vi "GUI_Single Button Pump.vi"() -> ()   [LabVIEW 2011] (continued)
                            n246 = Close Reference(reference=w680, error in (no error)=w679) -> (error out=w678:errorcluster)
                            n247 = invoke on="User Input Panel" class="SubPnl" method="Remove VI"(error in=w678) -> ()  [unwired: 2 in, 3 out]
                          }
                          frame Error {
                          }
                        }
                      }
                    }
                    n248 = call "MID-VAC Timer.vi"("TO sec (Start timer)"=1.0, "Action"=timerAction_typdef."Start Timer") -> ()  [unwired: 9 in, 1 out]
                  }
                  frame True {
                    # "when to is true\nand"
                    n249 = case shown="False" w682 {
                      tunnel: w683 -> [w689 _]
                      tunnel: [w687 w704] -> w684
                      tunnel: w681 -> [w685 w705]
                      frame False {
                        n250 = call "FindControlByName_VEPS.vi"("control name"="Op Out", "vi refnum"=w689) -> ("control refnum"=w691:refnum<vi>)  [unwired: 2 in, 1 out]
                        n251 = property class="Ctl"(reference=w691) -> ("Value"=w690:variant)  [unwired: 1 in, 2 out]
                        n252 = Variant To Data(type=op_typdef."Idle" ("Op Out"), Variant=w690) -> (data=w688:T24)  [unwired: 1 in, 1 out]
                        n253 = case shown="\"Continue to Wait\"" w688 {
                          tunnel: [w693 w699 "Idle\nMacro: Exit"] -> w687
                          tunnel: w685 -> [w694 w698 _]
                          frame "Idle", Default {
                            n254 = call "MID-VAC Timer.vi"("TO sec (Start timer)"=30.0, "Action"=timerAction_typdef."Start Timer") -> ()  [unwired: 9 in, 1 out]
                            n255 = Concatenate Strings("Main: BTL Sanity Check>>", w694) -> (w693:string)
                          }
                          frame "Continue to Wait" {
                            # "Continue to wait. Reset Timer"
                            n256 = call "MID-VAC Timer.vi"("TO sec (Start timer)"=30.0, "Action"=timerAction_typdef."Start Timer") -> ()  [unwired: 9 in, 1 out]
                            n257 = Concatenate Strings("Main: BTL Sanity Check>>", w698) -> (w699:string)
                          }
                          frame "Exit" {
                          }
                        }
                      }
                      frame True {
                        n258 = Concatenate Strings("Main: BTL Sanity Check>>", w705) -> (w704:string)
                      }
                    }
                  }
                }
                n259 = call "MID-VAC Timer.vi"("Action"=timerAction_typdef."Timer Running") -> ("TO"=w657:bool)  [unwired: 10 in]
                n260 = And(x=w652, y=w657) -> (x .and. y?=w656:bool)
                n261 = Concatenate Strings(w648, " Valve is NOT Closed. Perform corrective action.\nClick on continue to wait for some more time.\nClick Exit to abort GPM" ("message")) -> (w649:string)
                n262 = call "Generate TO event.vi"("Boolean"=w656, "message"=w649, "User Event in"=w659) -> ()  [unwired: 9 in]
              }
            }
          }
        }
        n263 = call <vilib>:"Add State(s) to Queue__jki_lib_state_machine.vi"("State(s) in Front (\"\")"=w623, "State(s) in (\"\")"=w617) -> ("States Out"=w628:string)  [unwired: 13 in]
      }
      frame "Main: TARGET Sanity Check" {
        # "Check if gate valve between COMP and M123 is Open"
        n264 = Unbundle By Name(w713) -> ("Chamber Selection.BTL"=w711:bool, "Chamber Selection.TARGET"=w712:bool, "Chamber Selection.BTL2"=w710:bool)
        n265 = case shown="True" w712 {
          tunnel: w718 -> [w721 w730]
          tunnel: w717 -> [_ w729]
          tunnel: [w721 w728] -> w716
          tunnel: w715 -> [_ w727]
          tunnel: ["" w726] -> w714
          tunnel: w713 -> [_ w725]
          tunnel: w711 -> [_ w723]
          tunnel: w710 -> [_ w722]
          tunnel: w709 -> [_ w724]
          frame False {
          }
          frame True {
            # "Check Conditions"
            n266 = case shown="\"BTL-TARGET,TARGET-BTL2\"" w724 {
              selector: w724 -> [_ w739]
              tunnel: w730 -> [w738 w756]
              tunnel: w729 -> [_ w755]
              tunnel: [w738 w753] -> w728
              tunnel: w727 -> [_ w750]
              tunnel: [w735 w744] -> w726
              tunnel: w725 -> [_ w742]
              tunnel: w723 -> [w732 _]
              tunnel: w722 -> [w736 _]
              frame "False", Default {
                # "COMP SELECTED?"
                n267 = Select(t="", s=w732, f="Main: TARGET Sanity Check>>BTL-TARGET") -> (s? t:f=w733:string)
                n268 = Select(t=w733, s=w736, f="Main: TARGET Sanity Check>>BTL-TARGET\nMain: TARGET Sanity Check>>TARGET-BTL2") -> (s? t:f=w735:string)
              }
              frame "BTL-TARGET,TARGET-BTL2" {
                w751 = Error_codes."003-Chamber Gate Valve Status" ("Error Codes")
                # "Event TAG"
                n269 = case shown="\"BTL-TARGET\"" w739 {
                  tunnel: [w758 w759 w760] -> w757
                  frame "False", Default {
                    w758 = T32[] [enum."No Action"] items=["No Action", "Is EC GPM Mode ON?", "Is EC GPM Mode Off?", "Is EC GVM Mode ON?", "Is EC GVM Off?", "Is  EC GPM or GVM Mode ON?", "Is LB GPM Mode ON?", "Is LB GPM Mode Off?", "Is LB GVM Mode ON?", "Is LB GVM Mode Off?", "Is  LB GPM or GVM Mode ON?", "Is M123 Turbo Gate Valve Opened? ", "Is M123 Turbo Gate Valve Closed?", "Is OAP Turbo Gate Valve Opened?", "Is OAP Turbo Gate Valve Closed?", "Is BTLTurbo Gate Valve Opened?", "Is BTL Turbo Gate Valve Closed?", "Is TARGET Turbo Gate Valve 1Opened?", "Is TARGET1 Turbo Gate Valve Closed?", "Is TARGET Turbo Gate Valve 2 Opened?", "Is TAREGT2 Turbo Gate Valve Closed?", "Is BTL2 Turbo Gate Valve Opened?", "Is BTL2 Turbo Gate Valve Closed?", "Is HPD Turbo Gate Valve Opened?", "Is HPD Turbo Gate Valve Closed?", "Is COMP to M123 gate Valve Opened?", "Is COMP to M123 Valve Closed?", "Is HPBD Gate Valve Opened?", "Is HPBD Gate Valve Closed?", "Is M123 to OAP gate valve opened?", "Is M123 to OAP gate valve closed?", "Is OAP to BLT gate valve opened?", "Is OAP to BTL Gate Valve Closed?", "Is BLT to TARGET gate valve opened?", "Is BTL to TARGET Gate Valve Closed?", "Is TARGET to BLT2 gate valve opened?", "Is TARGET to BTL2 Gate Valve Closed?", "Is BLT2 to HPD gate valve opened?", "Is BTL2 to HPD Gate Valve Closed?", "Is COMP at Atmospheric Pressure?", "Is M123 at Atmospheric Pressure?", "Is BeamDump at Atmospheric Pressure?", "Is OAP at Atmospheric Pressure?", "Is BLT at Atmospheric Pressure", "Is TARGET at Atmospheric Pressure?", "Is BLT2 at Atmospheric Pressure?", "Is HPD at Atmospheric Pressure?", "Is the EC Roughing Pump ON?", "Is the EC Roughing Pump OFF?", "Does the EC Roughing Pump have a fault?", "Is the LB Roughing Pump ON?", "Is the LB Roughing Pump Off?", "Does the LB Roughing Pump have a fault?", "Is the EC Backing Pump ON?", "Is the EC Backing Pump OFF?", "Is the LB Backing Pump ON?", "Is the LB Backing Pump OFF?", "Does the EC Backing Pump have a fault?", "Does the LB Backing Pump have a fault?", "Is the EC Backing Pipe at Atmospheric Pressure", "Is the LB Backing Pipe at Atmospheric Pressure", "Is the EC Backing Manifold at Atmospheric Pressure", "s the LB Backing Manifold at Atmospheric Pressure?", "Is the EC Roughing Pipe at Atmospheric Pressure", "Is the LB Roughing Pipe at Atmospheric Pressure?", "Is the EC Roughing Manifold at Atmospheric Pressure", "Is the LB Roughing Manifold at Atmospheric Pressure", "Is LB Backing Manifold Valve Opened?", "Is EC Backing Manifold Valve Opened?", "Is LB Roughing Manifold Valve Opened?", "Is EC Roughing Manifold Valve Opened?", "Is COMP Roughing Valve Opened?", "Is M123 Roughing Valve Opened?", "Is M123 Roughing Valve Closed?", "Is OAP Roughing Valve Opened?", "Is OAP Roughing Valve Closed?", "Is HPBD Roughing Valve Opened?", "Is HPBD Roughing Valve Closed?", "Is BTL Roughing Valve Opened?", "Is BTL Roughing Valve Closed?", "Is TARGET Roughing Valve Opened?", "Is TARGET Roughing Valve Closed?", "Is BTL2 Roughing Valve Opened?", "Is BTL2 Roughing Valve Closed?", "Is HPD Roughing Valve Opened?", "Is HPD Roughing Valve Closed?", "Is COMP Turbo Backing Valve Opened?", "Is M123 Turbo Backing Valve Opened", "Is HPBD Turbo Backing Valve Opened?", "Is OAP Turbo Backing Valve Opened?", "Is BTL Turbo Backing Valve Opened?", "Is TARGET1 Turbo Backing Valve Opened?", "Is TARGET2 Turbo Backing Valve Opened?", "Is BTL2 Turbo Backing Valve Opened?", "Is HPD Turbo Backing Valve Opened?", "Is M123 Backing at MID-VAC?", "Is OAP Backing at MID-VAC?", "Is TARGET1 Backing at MID-VAC?", "Is TARGET2 Backing at MID-VAC?", "Is BTL Backing at MID-VAC?", "Is BTL2 Backing at MID-VAC?", "Is HPD Backing at MID-VAC?", "Is M123 Turbo in Normal Operation", "Is COMP Turbo in Normal Operation", "Is OAP Turbo in Normal Operation", "Is BTL Turbo in Normal Operation", "Is TARGET1 Turbo in Normal Operation", "Is TARGET2 Turbo in Normal Operation", "Is BTL2 Turbo in Normal Operation", "Is HPD Turbo in Normal Operation", "Is M123 at MID-VAC?", "Is OAP at MID-VAC?", "Is COMP at MID-VAC?", "Is BTL at MID-VAC?", "Is TARGET at MID-VAC?", "Is BTL2 at MID-VAC?", "Is HPD at MID-VAC?"]
                  }
                  frame "TARGET-BTL2" {
                    w759 = T32[] [enum."Is TARGET to BTL2 Gate Valve Closed?"] items=["No Action", "Is EC GPM Mode ON?", "Is EC GPM Mode Off?", "Is EC GVM Mode ON?", "Is EC GVM Off?", "Is  EC GPM or GVM Mode ON?", "Is LB GPM Mode ON?", "Is LB GPM Mode Off?", "Is LB GVM Mode ON?", "Is LB GVM Mode Off?", "Is  LB GPM or GVM Mode ON?", "Is M123 Turbo Gate Valve Opened? ", "Is M123 Turbo Gate Valve Closed?", "Is OAP Turbo Gate Valve Opened?", "Is OAP Turbo Gate Valve Closed?", "Is BTLTurbo Gate Valve Opened?", "Is BTL Turbo Gate Valve Closed?", "Is TARGET Turbo Gate Valve 1Opened?", "Is TARGET1 Turbo Gate Valve Closed?", "Is TARGET Turbo Gate Valve 2 Opened?", "Is TAREGT2 Turbo Gate Valve Closed?", "Is BTL2 Turbo Gate Valve Opened?", "Is BTL2 Turbo Gate Valve Closed?", "Is HPD Turbo Gate Valve Opened?", "Is HPD Turbo Gate Valve Closed?", "Is COMP to M123 gate Valve Opened?", "Is COMP to M123 Valve Closed?", "Is HPBD Gate Valve Opened?", "Is HPBD Gate Valve Closed?", "Is M123 to OAP gate valve opened?", "Is M123 to OAP gate valve closed?", "Is OAP to BLT gate valve opened?", "Is OAP to BTL Gate Valve Closed?", "Is BLT to TARGET gate valve opened?", "Is BTL to TARGET Gate Valve Closed?", "Is TARGET to BLT2 gate valve opened?", "Is TARGET to BTL2 Gate Valve Closed?", "Is BLT2 to HPD gate valve opened?", "Is BTL2 to HPD Gate Valve Closed?", "Is COMP at Atmospheric Pressure?", "Is M123 at Atmospheric Pressure?", "Is BeamDump at Atmospheric Pressure?", "Is OAP at Atmospheric Pressure?", "Is BLT at Atmospheric Pressure", "Is TARGET at Atmospheric Pressure?", "Is BLT2 at Atmospheric Pressure?", "Is HPD at Atmospheric Pressure?", "Is the EC Roughing Pump ON?", "Is the EC Roughing Pump OFF?", "Does the EC Roughing Pump have a fault?", "Is the LB Roughing Pump ON?", "Is the LB Roughing Pump Off?", "Does the LB Roughing Pump have a fault?", "Is the EC Backing Pump ON?", "Is the EC Backing Pump OFF?", "Is the LB Backing Pump ON?", "Is the LB Backing Pump OFF?", "Does the EC Backing Pump have a fault?", "Does the LB Backing Pump have a fault?", "Is the EC Backing Pipe at Atmospheric Pressure", "Is the LB Backing Pipe at Atmospheric Pressure", "Is the EC Backing Manifold at Atmospheric Pressure", "s the LB Backing Manifold at Atmospheric Pressure?", "Is the EC Roughing Pipe at Atmospheric Pressure", "Is the LB Roughing Pipe at Atmospheric Pressure?", "Is the EC Roughing Manifold at Atmospheric Pressure", "Is the LB Roughing Manifold at Atmospheric Pressure", "Is LB Backing Manifold Valve Opened?", "Is EC Backing Manifold Valve Opened?", "Is LB Roughing Manifold Valve Opened?", "Is EC Roughing Manifold Valve Opened?", "Is COMP Roughing Valve Opened?", "Is M123 Roughing Valve Opened?", "Is M123 Roughing Valve Closed?", "Is OAP Roughing Valve Opened?", "Is OAP Roughing Valve Closed?", "Is HPBD Roughing Valve Opened?", "Is HPBD Roughing Valve Closed?", "Is BTL Roughing Valve Opened?", "Is BTL Roughing Valve Closed?", "Is TARGET Roughing Valve Opened?", "Is TARGET Roughing Valve Closed?", "Is BTL2 Roughing Valve Opened?", "Is BTL2 Roughing Valve Closed?", "Is HPD Roughing Valve Opened?", "Is HPD Roughing Valve Closed?", "Is COMP Turbo Backing Valve Opened?", "Is M123 Turbo Backing Valve Opened", "Is HPBD Turbo Backing Valve Opened?", "Is OAP Turbo Backing Valve Opened?", "Is BTL Turbo Backing Valve Opened?", "Is TARGET1 Turbo Backing Valve Opened?", "Is TARGET2 Turbo Backing Valve Opened?", "Is BTL2 Turbo Backing Valve Opened?", "Is HPD Turbo Backing Valve Opened?", "Is M123 Backing at MID-VAC?", "Is OAP Backing at MID-VAC?", "Is TARGET1 Backing at MID-VAC?", "Is TARGET2 Backing at MID-VAC?", "Is BTL Backing at MID-VAC?", "Is BTL2 Backing at MID-VAC?", "Is HPD Backing at MID-VAC?", "Is M123 Turbo in Normal Operation", "Is COMP Turbo in Normal Operation", "Is OAP Turbo in Normal Operation", "Is BTL Turbo in Normal Operation", "Is TARGET1 Turbo in Normal Operation", "Is TARGET2 Turbo in Normal Operation", "Is BTL2 Turbo in Normal Operation", "Is HPD Turbo in Normal Operation", "Is M123 at MID-VAC?", "Is OAP at MID-VAC?", "Is COMP at MID-VAC?", "Is BTL at MID-VAC?", "Is TARGET at MID-VAC?", "Is BTL2 at MID-VAC?", "Is HPD at MID-VAC?"]
                  }
                  frame "BTL-TARGET" {
                    w760 = T32[] [enum."Is BTL to TARGET Gate Valve Closed?"] items=["No Action", "Is EC GPM Mode ON?", "Is EC GPM Mode Off?", "Is EC GVM Mode ON?", "Is EC GVM Off?", "Is  EC GPM or GVM Mode ON?", "Is LB GPM Mode ON?", "Is LB GPM Mode Off?", "Is LB GVM Mode ON?", "Is LB GVM Mode Off?", "Is  LB GPM or GVM Mode ON?", "Is M123 Turbo Gate Valve Opened? ", "Is M123 Turbo Gate Valve Closed?", "Is OAP Turbo Gate Valve Opened?", "Is OAP Turbo Gate Valve Closed?", "Is BTLTurbo Gate Valve Opened?", "Is BTL Turbo Gate Valve Closed?", "Is TARGET Turbo Gate Valve 1Opened?", "Is TARGET1 Turbo Gate Valve Closed?", "Is TARGET Turbo Gate Valve 2 Opened?", "Is TAREGT2 Turbo Gate Valve Closed?", "Is BTL2 Turbo Gate Valve Opened?", "Is BTL2 Turbo Gate Valve Closed?", "Is HPD Turbo Gate Valve Opened?", "Is HPD Turbo Gate Valve Closed?", "Is COMP to M123 gate Valve Opened?", "Is COMP to M123 Valve Closed?", "Is HPBD Gate Valve Opened?", "Is HPBD Gate Valve Closed?", "Is M123 to OAP gate valve opened?", "Is M123 to OAP gate valve closed?", "Is OAP to BLT gate valve opened?", "Is OAP to BTL Gate Valve Closed?", "Is BLT to TARGET gate valve opened?", "Is BTL to TARGET Gate Valve Closed?", "Is TARGET to BLT2 gate valve opened?", "Is TARGET to BTL2 Gate Valve Closed?", "Is BLT2 to HPD gate valve opened?", "Is BTL2 to HPD Gate Valve Closed?", "Is COMP at Atmospheric Pressure?", "Is M123 at Atmospheric Pressure?", "Is BeamDump at Atmospheric Pressure?", "Is OAP at Atmospheric Pressure?", "Is BLT at Atmospheric Pressure", "Is TARGET at Atmospheric Pressure?", "Is BLT2 at Atmospheric Pressure?", "Is HPD at Atmospheric Pressure?", "Is the EC Roughing Pump ON?", "Is the EC Roughing Pump OFF?", "Does the EC Roughing Pump have a fault?", "Is the LB Roughing Pump ON?", "Is the LB Roughing Pump Off?", "Does the LB Roughing Pump have a fault?", "Is the EC Backing Pump ON?", "Is the EC Backing Pump OFF?", "Is the LB Backing Pump ON?", "Is the LB Backing Pump OFF?", "Does the EC Backing Pump have a fault?", "Does the LB Backing Pump have a fault?", "Is the EC Backing Pipe at Atmospheric Pressure", "Is the LB Backing Pipe at Atmospheric Pressure", "Is the EC Backing Manifold at Atmospheric Pressure", "s the LB Backing Manifold at Atmospheric Pressure?", "Is the EC Roughing Pipe at Atmospheric Pressure", "Is the LB Roughing Pipe at Atmospheric Pressure?", "Is the EC Roughing Manifold at Atmospheric Pressure", "Is the LB Roughing Manifold at Atmospheric Pressure", "Is LB Backing Manifold Valve Opened?", "Is EC Backing Manifold Valve Opened?", "Is LB Roughing Manifold Valve Opened?", "Is EC Roughing Manifold Valve Opened?", "Is COMP Roughing Valve Opened?", "Is M123 Roughing Valve Opened?", "Is M123 Roughing Valve Closed?", "Is OAP Roughing Valve Opened?", "Is OAP Roughing Valve Closed?", "Is HPBD Roughing Valve Opened?", "Is HPBD Roughing Valve Closed?", "Is BTL Roughing Valve Opened?", "Is BTL Roughing Valve Closed?", "Is TARGET Roughing Valve Opened?", "Is TARGET Roughing Valve Closed?", "Is BTL2 Roughing Valve Opened?", "Is BTL2 Roughing Valve Closed?", "Is HPD Roughing Valve Opened?", "Is HPD Roughing Valve Closed?", "Is COMP Turbo Backing Valve Opened?", "Is M123 Turbo Backing Valve Opened", "Is HPBD Turbo Backing Valve Opened?", "Is OAP Turbo Backing Valve Opened?", "Is BTL Turbo Backing Valve Opened?", "Is TARGET1 Turbo Backing Valve Opened?", "Is TARGET2 Turbo Backing Valve Opened?", "Is BTL2 Turbo Backing Valve Opened?", "Is HPD Turbo Backing Valve Opened?", "Is M123 Backing at MID-VAC?", "Is OAP Backing at MID-VAC?", "Is TARGET1 Backing at MID-VAC?", "Is TARGET2 Backing at MID-VAC?", "Is BTL Backing at MID-VAC?", "Is BTL2 Backing at MID-VAC?", "Is HPD Backing at MID-VAC?", "Is M123 Turbo in Normal Operation", "Is COMP Turbo in Normal Operation", "Is OAP Turbo in Normal Operation", "Is BTL Turbo in Normal Operation", "Is TARGET1 Turbo in Normal Operation", "Is TARGET2 Turbo in Normal Operation", "Is BTL2 Turbo in Normal Operation", "Is HPD Turbo in Normal Operation", "Is M123 at MID-VAC?", "Is OAP at MID-VAC?", "Is COMP at MID-VAC?", "Is BTL at MID-VAC?", "Is TARGET at MID-VAC?", "Is BTL2 at MID-VAC?", "Is HPD at MID-VAC?"]
                  }
                }
                n270 = call "GetAction.vi"("Check Condition"=w751, "Query Array"=w757, "error in (no error)"=w756) -> ("Status Array Out"=w752:string[], "Generate Event?"=w743:bool, "error out"=w754:errorcluster)  [unwired: 7 in, 3 out]
                n271 = Unbundle By Name(w742) -> ("VI Refnum"=w746:refnum<vi>)
                n272 = call "Generate User Event.vi"("Add(t)/Remove(f) Event"=w743, "error in (no error)"=w754, "User Event in"=w755, "Status Array In"=w752, "Error Codes"=w751) -> ("error out"=w753:errorcluster)  [unwired: 5 in, 1 out]
                n273 = Not A Number/Path/Refnum?(number/path/refnum=w746) -> (NaN/Path/Refnum?=w745:bool)
                n274 = case shown="True" w743 {
                  tunnel: ["" w775] -> w744
                  tunnel: w746 -> [w764 w774]
                  tunnel: w745 -> [w765 w773]
                  tunnel: w739 -> [_ w772]
                  frame False {
                    n275 = case shown="True" w765 {
                      tunnel: w764 -> [_ w768]
                      frame False {
                      }
                      frame True {
                        n276 = invoke class="VI" method="Abort VI"(reference=w768) -> (reference out=w766:refnum<vi>, error out=w767:errorcluster)  [unwired: 2 in, 1 out]
                        n277 = case shown="No Error" w767 {
                          selector: w767 -> [w770 _]
                          tunnel: w766 -> [w771 _]
                          frame No Error {
                            n278 = Close Reference(reference=w771, error in (no error)=w770) -> (error out=w769:errorcluster)
                            n279 = invoke on="User Input Panel" class="SubPnl" method="Remove VI"(error in=w769) -> ()  [unwired: 2 in, 3 out]
                          }
                          frame Error {
                          }
                        }
                      }
                    }
                    n280 = call "MID-VAC Timer.vi"("TO sec (Start timer)"=1.0, "Action"=timerAction_typdef."Start Timer") -> ()  [unwired: 9 in, 1 out]
                  }
                  frame True {
                    # "when to is true\nand"
                    n281 = case shown="True" w773 {
                      tunnel: w774 -> [w780 _]
                      tunnel: [w778 w795] -> w775
                      tunnel: w772 -> [w776 w796]
                      frame False {
                        n282 = call "FindControlByName_VEPS.vi"("control name"="Op Out", "vi refnum"=w780) -> ("control refnum"=w782:refnum<vi>)  [unwired: 2 in, 1 out]
                        n283 = property class="Ctl"(reference=w782) -> ("Value"=w781:variant)  [unwired: 1 in, 2 out]
                        n284 = Variant To Data(type=op_typdef."Idle" ("Op Out"), Variant=w781) -> (data=w779:T24)  [unwired: 1 in, 1 out]
                        n285 = case shown="\"Idle\", Default" w779 {
                          tunnel: [w784 w790 "Idle\nMacro: Exit"] -> w778
                          tunnel: w776 -> [w785 w789 _]
                          frame "Idle", Default {
                            n286 = call "MID-VAC Timer.vi"("TO sec (Start timer)"=30.0, "Action"=timerAction_typdef."Start Timer") -> ()  [unwired: 9 in, 1 out]
                            n287 = Concatenate Strings("Main: TARGET Sanity Check>>", w785) -> (w784:string)
                          }
                          frame "Continue to Wait" {
                            # "Continue to wait. Reset Timer"
                            n288 = call "MID-VAC Timer.vi"("TO sec (Start timer)"=30.0, "Action"=timerAction_typdef."Start Timer") -> ()  [unwired: 9 in, 1 out]
                            n289 = Concatenate Strings("Main: TARGET Sanity Check>>", w789) -> (w790:string)
                          }
                          frame "Exit" {
                          }
                        }
                      }
                      frame True {
                        n290 = Concatenate Strings("Main: TARGET Sanity Check>>", w796) -> (w795:string)
                      }
                    }
                  }
                }
                n291 = call "MID-VAC Timer.vi"("Action"=timerAction_typdef."Timer Running") -> ("TO"=w748:bool)  [unwired: 10 in]
                n292 = And(x=w743, y=w748) -> (x .and. y?=w747:bool)
                n293 = Concatenate Strings(w739, " Valve is NOT Closed. Perform corrective action.\nClick on continue to wait for some more time.\nClick Exit to abort GPM" ("message")) -> (w740:string)
                n294 = call "Generate TO event.vi"("Boolean"=w747, "message"=w740, "User Event in"=w750) -> ()  [unwired: 9 in]
              }
            }
          }
        }
        n295 = call <vilib>:"Add State(s) to Queue__jki_lib_state_machine.vi"("State(s) in Front (\"\")"=w714, "State(s) in (\"\")"=w708) -> ("States Out"=w719:string)  [unwired: 13 in]
      }
      frame "Main: BTL2 Sanity Check" {
        # "Check if gate valve between COMP and M123 is Open"
        n296 = Unbundle By Name(w804) -> ("Chamber Selection.TARGET"=w802:bool, "Chamber Selection.BTL2"=w803:bool, "Chamber Selection.HPD"=w801:bool)
        n297 = case shown="True" w803 {
          tunnel: w809 -> [w812 w821]
          tunnel: w808 -> [_ w820]
          tunnel: [w812 w819] -> w807
          tunnel: w806 -> [_ w818]
          tunnel: ["" w817] -> w805
          tunnel: w804 -> [_ w816]
          tunnel: w802 -> [_ w814]
          tunnel: w801 -> [_ w813]
          tunnel: w800 -> [_ w815]
          frame False {
          }
          frame True {
            # "Check Conditions"
            n298 = case shown="\"BTL2-HPD,TARGET-BTL2\"" w815 {
              selector: w815 -> [_ w830]
              tunnel: w821 -> [w829 w847]
              tunnel: w820 -> [_ w846]
              tunnel: [w829 w844] -> w819
              tunnel: w818 -> [_ w841]
              tunnel: [w826 w835] -> w817
              tunnel: w816 -> [_ w833]
              tunnel: w814 -> [w823 _]
              tunnel: w813 -> [w827 _]
              frame "False", Default {
                # "COMP SELECTED?"
                n299 = Select(t="", s=w823, f="Main: BTL2 Sanity Check>>TARGET-BTL2") -> (s? t:f=w824:string)
                n300 = Select(t=w824, s=w827, f="Main: BTL2 Sanity Check>>TARGET-BTL2\nMain: BTL2 Sanity Check>>BTL2-HPD") -> (s? t:f=w826:string)
              }
              frame "BTL2-HPD,TARGET-BTL2" {
                w842 = Error_codes."003-Chamber Gate Valve Status" ("Error Codes")
                # "Event TAG"
                n301 = case shown="\"BTL2-HPD\"" w830 {
                  tunnel: [w849 w850 w851] -> w848
                  frame "False", Default {
                    w849 = T32[] [enum."No Action"] items=["No Action", "Is EC GPM Mode ON?", "Is EC GPM Mode Off?", "Is EC GVM Mode ON?", "Is EC GVM Off?", "Is  EC GPM or GVM Mode ON?", "Is LB GPM Mode ON?", "Is LB GPM Mode Off?", "Is LB GVM Mode ON?", "Is LB GVM Mode Off?", "Is  LB GPM or GVM Mode ON?", "Is M123 Turbo Gate Valve Opened? ", "Is M123 Turbo Gate Valve Closed?", "Is OAP Turbo Gate Valve Opened?", "Is OAP Turbo Gate Valve Closed?", "Is BTLTurbo Gate Valve Opened?", "Is BTL Turbo Gate Valve Closed?", "Is TARGET Turbo Gate Valve 1Opened?", "Is TARGET1 Turbo Gate Valve Closed?", "Is TARGET Turbo Gate Valve 2 Opened?", "Is TAREGT2 Turbo Gate Valve Closed?", "Is BTL2 Turbo Gate Valve Opened?", "Is BTL2 Turbo Gate Valve Closed?", "Is HPD Turbo Gate Valve Opened?", "Is HPD Turbo Gate Valve Closed?", "Is COMP to M123 gate Valve Opened?", "Is COMP to M123 Valve Closed?", "Is HPBD Gate Valve Opened?", "Is HPBD Gate Valve Closed?", "Is M123 to OAP gate valve opened?", "Is M123 to OAP gate valve closed?", "Is OAP to BLT gate valve opened?", "Is OAP to BTL Gate Valve Closed?", "Is BLT to TARGET gate valve opened?", "Is BTL to TARGET Gate Valve Closed?", "Is TARGET to BLT2 gate valve opened?", "Is TARGET to BTL2 Gate Valve Closed?", "Is BLT2 to HPD gate valve opened?", "Is BTL2 to HPD Gate Valve Closed?", "Is COMP at Atmospheric Pressure?", "Is M123 at Atmospheric Pressure?", "Is BeamDump at Atmospheric Pressure?", "Is OAP at Atmospheric Pressure?", "Is BLT at Atmospheric Pressure", "Is TARGET at Atmospheric Pressure?", "Is BLT2 at Atmospheric Pressure?", "Is HPD at Atmospheric Pressure?", "Is the EC Roughing Pump ON?", "Is the EC Roughing Pump OFF?", "Does the EC Roughing Pump have a fault?", "Is the LB Roughing Pump ON?", "Is the LB Roughing Pump Off?", "Does the LB Roughing Pump have a fault?", "Is the EC Backing Pump ON?", "Is the EC Backing Pump OFF?", "Is the LB Backing Pump ON?", "Is the LB Backing Pump OFF?", "Does the EC Backing Pump have a fault?", "Does the LB Backing Pump have a fault?", "Is the EC Backing Pipe at Atmospheric Pressure", "Is the LB Backing Pipe at Atmospheric Pressure", "Is the EC Backing Manifold at Atmospheric Pressure", "s the LB Backing Manifold at Atmospheric Pressure?", "Is the EC Roughing Pipe at Atmospheric Pressure", "Is the LB Roughing Pipe at Atmospheric Pressure?", "Is the EC Roughing Manifold at Atmospheric Pressure", "Is the LB Roughing Manifold at Atmospheric Pressure", "Is LB Backing Manifold Valve Opened?", "Is EC Backing Manifold Valve Opened?", "Is LB Roughing Manifold Valve Opened?", "Is EC Roughing Manifold Valve Opened?", "Is COMP Roughing Valve Opened?", "Is M123 Roughing Valve Opened?", "Is M123 Roughing Valve Closed?", "Is OAP Roughing Valve Opened?", "Is OAP Roughing Valve Closed?", "Is HPBD Roughing Valve Opened?", "Is HPBD Roughing Valve Closed?", "Is BTL Roughing Valve Opened?", "Is BTL Roughing Valve Closed?", "Is TARGET Roughing Valve Opened?", "Is TARGET Roughing Valve Closed?", "Is BTL2 Roughing Valve Opened?", "Is BTL2 Roughing Valve Closed?", "Is HPD Roughing Valve Opened?", "Is HPD Roughing Valve Closed?", "Is COMP Turbo Backing Valve Opened?", "Is M123 Turbo Backing Valve Opened", "Is HPBD Turbo Backing Valve Opened?", "Is OAP Turbo Backing Valve Opened?", "Is BTL Turbo Backing Valve Opened?", "Is TARGET1 Turbo Backing Valve Opened?", "Is TARGET2 Turbo Backing Valve Opened?", "Is BTL2 Turbo Backing Valve Opened?", "Is HPD Turbo Backing Valve Opened?", "Is M123 Backing at MID-VAC?", "Is OAP Backing at MID-VAC?", "Is TARGET1 Backing at MID-VAC?", "Is TARGET2 Backing at MID-VAC?", "Is BTL Backing at MID-VAC?", "Is BTL2 Backing at MID-VAC?", "Is HPD Backing at MID-VAC?", "Is M123 Turbo in Normal Operation", "Is COMP Turbo in Normal Operation", "Is OAP Turbo in Normal Operation", "Is BTL Turbo in Normal Operation", "Is TARGET1 Turbo in Normal Operation", "Is TARGET2 Turbo in Normal Operation", "Is BTL2 Turbo in Normal Operation", "Is HPD Turbo in Normal Operation", "Is M123 at MID-VAC?", "Is OAP at MID-VAC?", "Is COMP at MID-VAC?", "Is BTL at MID-VAC?", "Is TARGET at MID-VAC?", "Is BTL2 at MID-VAC?", "Is HPD at MID-VAC?"]
                  }
                  frame "TARGET-BTL2" {
                    w850 = T32[] [enum."Is TARGET to BTL2 Gate Valve Closed?"] items=["No Action", "Is EC GPM Mode ON?", "Is EC GPM Mode Off?", "Is EC GVM Mode ON?", "Is EC GVM Off?", "Is  EC GPM or GVM Mode ON?", "Is LB GPM Mode ON?", "Is LB GPM Mode Off?", "Is LB GVM Mode ON?", "Is LB GVM Mode Off?", "Is  LB GPM or GVM Mode ON?", "Is M123 Turbo Gate Valve Opened? ", "Is M123 Turbo Gate Valve Closed?", "Is OAP Turbo Gate Valve Opened?", "Is OAP Turbo Gate Valve Closed?", "Is BTLTurbo Gate Valve Opened?", "Is BTL Turbo Gate Valve Closed?", "Is TARGET Turbo Gate Valve 1Opened?", "Is TARGET1 Turbo Gate Valve Closed?", "Is TARGET Turbo Gate Valve 2 Opened?", "Is TAREGT2 Turbo Gate Valve Closed?", "Is BTL2 Turbo Gate Valve Opened?", "Is BTL2 Turbo Gate Valve Closed?", "Is HPD Turbo Gate Valve Opened?", "Is HPD Turbo Gate Valve Closed?", "Is COMP to M123 gate Valve Opened?", "Is COMP to M123 Valve Closed?", "Is HPBD Gate Valve Opened?", "Is HPBD Gate Valve Closed?", "Is M123 to OAP gate valve opened?", "Is M123 to OAP gate valve closed?", "Is OAP to BLT gate valve opened?", "Is OAP to BTL Gate Valve Closed?", "Is BLT to TARGET gate valve opened?", "Is BTL to TARGET Gate Valve Closed?", "Is TARGET to BLT2 gate valve opened?", "Is TARGET to BTL2 Gate Valve Closed?", "Is BLT2 to HPD gate valve opened?", "Is BTL2 to HPD Gate Valve Closed?", "Is COMP at Atmospheric Pressure?", "Is M123 at Atmospheric Pressure?", "Is BeamDump at Atmospheric Pressure?", "Is OAP at Atmospheric Pressure?", "Is BLT at Atmospheric Pressure", "Is TARGET at Atmospheric Pressure?", "Is BLT2 at Atmospheric Pressure?", "Is HPD at Atmospheric Pressure?", "Is the EC Roughing Pump ON?", "Is the EC Roughing Pump OFF?", "Does the EC Roughing Pump have a fault?", "Is the LB Roughing Pump ON?", "Is the LB Roughing Pump Off?", "Does the LB Roughing Pump have a fault?", "Is the EC Backing Pump ON?", "Is the EC Backing Pump OFF?", "Is the LB Backing Pump ON?", "Is the LB Backing Pump OFF?", "Does the EC Backing Pump have a fault?", "Does the LB Backing Pump have a fault?", "Is the EC Backing Pipe at Atmospheric Pressure", "Is the LB Backing Pipe at Atmospheric Pressure", "Is the EC Backing Manifold at Atmospheric Pressure", "s the LB Backing Manifold at Atmospheric Pressure?", "Is the EC Roughing Pipe at Atmospheric Pressure", "Is the LB Roughing Pipe at Atmospheric Pressure?", "Is the EC Roughing Manifold at Atmospheric Pressure", "Is the LB Roughing Manifold at Atmospheric Pressure", "Is LB Backing Manifold Valve Opened?", "Is EC Backing Manifold Valve Opened?", "Is LB Roughing Manifold Valve Opened?", "Is EC Roughing Manifold Valve Opened?", "Is COMP Roughing Valve Opened?", "Is M123 Roughing Valve Opened?", "Is M123 Roughing Valve Closed?", "Is OAP Roughing Valve Opened?", "Is OAP Roughing Valve Closed?", "Is HPBD Roughing Valve Opened?", "Is HPBD Roughing Valve Closed?", "Is BTL Roughing Valve Opened?", "Is BTL Roughing Valve Closed?", "Is TARGET Roughing Valve Opened?", "Is TARGET Roughing Valve Closed?", "Is BTL2 Roughing Valve Opened?", "Is BTL2 Roughing Valve Closed?", "Is HPD Roughing Valve Opened?", "Is HPD Roughing Valve Closed?", "Is COMP Turbo Backing Valve Opened?", "Is M123 Turbo Backing Valve Opened", "Is HPBD Turbo Backing Valve Opened?", "Is OAP Turbo Backing Valve Opened?", "Is BTL Turbo Backing Valve Opened?", "Is TARGET1 Turbo Backing Valve Opened?", "Is TARGET2 Turbo Backing Valve Opened?", "Is BTL2 Turbo Backing Valve Opened?", "Is HPD Turbo Backing Valve Opened?", "Is M123 Backing at MID-VAC?", "Is OAP Backing at MID-VAC?", "Is TARGET1 Backing at MID-VAC?", "Is TARGET2 Backing at MID-VAC?", "Is BTL Backing at MID-VAC?", "Is BTL2 Backing at MID-VAC?", "Is HPD Backing at MID-VAC?", "Is M123 Turbo in Normal Operation", "Is COMP Turbo in Normal Operation", "Is OAP Turbo in Normal Operation", "Is BTL Turbo in Normal Operation", "Is TARGET1 Turbo in Normal Operation", "Is TARGET2 Turbo in Normal Operation", "Is BTL2 Turbo in Normal Operation", "Is HPD Turbo in Normal Operation", "Is M123 at MID-VAC?", "Is OAP at MID-VAC?", "Is COMP at MID-VAC?", "Is BTL at MID-VAC?", "Is TARGET at MID-VAC?", "Is BTL2 at MID-VAC?", "Is HPD at MID-VAC?"]
                  }
                  frame "BTL2-HPD" {
                    w851 = T32[] [enum."Is BTL2 to HPD Gate Valve Closed?"] items=["No Action", "Is EC GPM Mode ON?", "Is EC GPM Mode Off?", "Is EC GVM Mode ON?", "Is EC GVM Off?", "Is  EC GPM or GVM Mode ON?", "Is LB GPM Mode ON?", "Is LB GPM Mode Off?", "Is LB GVM Mode ON?", "Is LB GVM Mode Off?", "Is  LB GPM or GVM Mode ON?", "Is M123 Turbo Gate Valve Opened? ", "Is M123 Turbo Gate Valve Closed?", "Is OAP Turbo Gate Valve Opened?", "Is OAP Turbo Gate Valve Closed?", "Is BTLTurbo Gate Valve Opened?", "Is BTL Turbo Gate Valve Closed?", "Is TARGET Turbo Gate Valve 1Opened?", "Is TARGET1 Turbo Gate Valve Closed?", "Is TARGET Turbo Gate Valve 2 Opened?", "Is TAREGT2 Turbo Gate Valve Closed?", "Is BTL2 Turbo Gate Valve Opened?", "Is BTL2 Turbo Gate Valve Closed?", "Is HPD Turbo Gate Valve Opened?", "Is HPD Turbo Gate Valve Closed?", "Is COMP to M123 gate Valve Opened?", "Is COMP to M123 Valve Closed?", "Is HPBD Gate Valve Opened?", "Is HPBD Gate Valve Closed?", "Is M123 to OAP gate valve opened?", "Is M123 to OAP gate valve closed?", "Is OAP to BLT gate valve opened?", "Is OAP to BTL Gate Valve Closed?", "Is BLT to TARGET gate valve opened?", "Is BTL to TARGET Gate Valve Closed?", "Is TARGET to BLT2 gate valve opened?", "Is TARGET to BTL2 Gate Valve Closed?", "Is BLT2 to HPD gate valve opened?", "Is BTL2 to HPD Gate Valve Closed?", "Is COMP at Atmospheric Pressure?", "Is M123 at Atmospheric Pressure?", "Is BeamDump at Atmospheric Pressure?", "Is OAP at Atmospheric Pressure?", "Is BLT at Atmospheric Pressure", "Is TARGET at Atmospheric Pressure?", "Is BLT2 at Atmospheric Pressure?", "Is HPD at Atmospheric Pressure?", "Is the EC Roughing Pump ON?", "Is the EC Roughing Pump OFF?", "Does the EC Roughing Pump have a fault?", "Is the LB Roughing Pump ON?", "Is the LB Roughing Pump Off?", "Does the LB Roughing Pump have a fault?", "Is the EC Backing Pump ON?", "Is the EC Backing Pump OFF?", "Is the LB Backing Pump ON?", "Is the LB Backing Pump OFF?", "Does the EC Backing Pump have a fault?", "Does the LB Backing Pump have a fault?", "Is the EC Backing Pipe at Atmospheric Pressure", "Is the LB Backing Pipe at Atmospheric Pressure", "Is the EC Backing Manifold at Atmospheric Pressure", "s the LB Backing Manifold at Atmospheric Pressure?", "Is the EC Roughing Pipe at Atmospheric Pressure", "Is the LB Roughing Pipe at Atmospheric Pressure?", "Is the EC Roughing Manifold at Atmospheric Pressure", "Is the LB Roughing Manifold at Atmospheric Pressure", "Is LB Backing Manifold Valve Opened?", "Is EC Backing Manifold Valve Opened?", "Is LB Roughing Manifold Valve Opened?", "Is EC Roughing Manifold Valve Opened?", "Is COMP Roughing Valve Opened?", "Is M123 Roughing Valve Opened?", "Is M123 Roughing Valve Closed?", "Is OAP Roughing Valve Opened?", "Is OAP Roughing Valve Closed?", "Is HPBD Roughing Valve Opened?", "Is HPBD Roughing Valve Closed?", "Is BTL Roughing Valve Opened?", "Is BTL Roughing Valve Closed?", "Is TARGET Roughing Valve Opened?", "Is TARGET Roughing Valve Closed?", "Is BTL2 Roughing Valve Opened?", "Is BTL2 Roughing Valve Closed?", "Is HPD Roughing Valve Opened?", "Is HPD Roughing Valve Closed?", "Is COMP Turbo Backing Valve Opened?", "Is M123 Turbo Backing Valve Opened", "Is HPBD Turbo Backing Valve Opened?", "Is OAP Turbo Backing Valve Opened?", "Is BTL Turbo Backing Valve Opened?", "Is TARGET1 Turbo Backing Valve Opened?", "Is TARGET2 Turbo Backing Valve Opened?", "Is BTL2 Turbo Backing Valve Opened?", "Is HPD Turbo Backing Valve Opened?", "Is M123 Backing at MID-VAC?", "Is OAP Backing at MID-VAC?", "Is TARGET1 Backing at MID-VAC?", "Is TARGET2 Backing at MID-VAC?", "Is BTL Backing at MID-VAC?", "Is BTL2 Backing at MID-VAC?", "Is HPD Backing at MID-VAC?", "Is M123 Turbo in Normal Operation", "Is COMP Turbo in Normal Operation", "Is OAP Turbo in Normal Operation", "Is BTL Turbo in Normal Operation", "Is TARGET1 Turbo in Normal Operation", "Is TARGET2 Turbo in Normal Operation", "Is BTL2 Turbo in Normal Operation", "Is HPD Turbo in Normal Operation", "Is M123 at MID-VAC?", "Is OAP at MID-VAC?", "Is COMP at MID-VAC?", "Is BTL at MID-VAC?", "Is TARGET at MID-VAC?", "Is BTL2 at MID-VAC?", "Is HPD at MID-VAC?"]
                  }
                }
                n302 = call "GetAction.vi"("Check Condition"=w842, "Query Array"=w848, "error in (no error)"=w847) -> ("Status Array Out"=w843:string[], "Generate Event?"=w834:bool, "error out"=w845:errorcluster)  [unwired: 7 in, 3 out]
                n303 = Unbundle By Name(w833) -> ("VI Refnum"=w837:refnum<vi>)
                n304 = call "Generate User Event.vi"("Add(t)/Remove(f) Event"=w834, "error in (no error)"=w845, "User Event in"=w846, "Status Array In"=w843, "Error Codes"=w842) -> ("error out"=w844:errorcluster)  [unwired: 5 in, 1 out]
                n305 = Not A Number/Path/Refnum?(number/path/refnum=w837) -> (NaN/Path/Refnum?=w836:bool)
                n306 = case shown="True" w834 {
                  tunnel: ["" w866] -> w835
                  tunnel: w837 -> [w855 w865]
                  tunnel: w836 -> [w856 w864]
                  tunnel: w830 -> [_ w863]
                  frame False {
                    n307 = case shown="True" w856 {
                      tunnel: w855 -> [_ w859]
                      frame False {
                      }
                      frame True {
                        n308 = invoke class="VI" method="Abort VI"(reference=w859) -> (reference out=w857:refnum<vi>, error out=w858:errorcluster)  [unwired: 2 in, 1 out]
                        n309 = case shown="No Error" w858 {
                          selector: w858 -> [w861 _]
                          tunnel: w857 -> [w862 _]
                          frame No Error {
                            n310 = Close Reference(reference=w862, error in (no error)=w861) -> (error out=w860:errorcluster)
                            n311 = invoke on="User Input Panel" class="SubPnl" method="Remove VI"(error in=w860) -> ()  [unwired: 2 in, 3 out]
                          }
                          frame Error {
                          }
                        }
                      }
                    }
                    n312 = call "MID-VAC Timer.vi"("TO sec (Start timer)"=1.0, "Action"=timerAction_typdef."Start Timer") -> ()  [unwired: 9 in, 1 out]
                  }
                  frame True {
                    # "when to is true\nand"
                    n313 = case shown="False" w864 {
                      tunnel: w865 -> [w871 _]
                      tunnel: [w869 w886] -> w866
                      tunnel: w863 -> [w867 w887]
                      frame False {
                        n314 = call "FindControlByName_VEPS.vi"("control name"="Op Out", "vi refnum"=w871) -> ("control refnum"=w873:refnum<vi>)  [unwired: 2 in, 1 out]
                        n315 = property class="Ctl"(reference=w873) -> ("Value"=w872:variant)  [unwired: 1 in, 2 out]
                        n316 = Variant To Data(type=op_typdef."Idle" ("Op Out"), Variant=w872) -> (data=w870:T24)  [unwired: 1 in, 1 out]
                        n317 = case shown="\"Idle\", Default" w870 {
                          tunnel: [w875 w881 "Idle\nMacro: Exit"] -> w869
                          tunnel: w867 -> [w876 w880 _]
                          frame "Idle", Default {
                            n318 = call "MID-VAC Timer.vi"("TO sec (Start timer)"=30.0, "Action"=timerAction_typdef."Start Timer") -> ()  [unwired: 9 in, 1 out]
                            n319 = Concatenate Strings("Main: BTL2 Sanity Check>>", w876) -> (w875:string)
                          }
                          frame "Continue to Wait" {
                            # "Continue to wait. Reset Timer"
                            n320 = call "MID-VAC Timer.vi"("TO sec (Start timer)"=30.0, "Action"=timerAction_typdef."Start Timer") -> ()  [unwired: 9 in, 1 out]
                            n321 = Concatenate Strings("Main: BTL2 Sanity Check>>", w880) -> (w881:string)
                          }
                          frame "Exit" {
                          }
                        }
                      }
                      frame True {
                        n322 = Concatenate Strings("Main: BTL2 Sanity Check>>", w887) -> (w886:string)
                      }
                    }
                  }
                }
                n323 = call "MID-VAC Timer.vi"("Action"=timerAction_typdef."Timer Running") -> ("TO"=w839:bool)  [unwired: 10 in]
                n324 = And(x=w834, y=w839) -> (x .and. y?=w838:bool)
                n325 = Concatenate Strings(w830, " Valve is NOT Closed. Perform corrective action.\nClick on continue to wait for some more time.\nClick Exit to abort GPM" ("message")) -> (w831:string)
                n326 = call "Generate TO event.vi"("Boolean"=w838, "message"=w831, "User Event in"=w841) -> ()  [unwired: 9 in]
              }
            }
          }
        }
        n327 = call <vilib>:"Add State(s) to Queue__jki_lib_state_machine.vi"("State(s) in Front (\"\")"=w805, "State(s) in (\"\")"=w799) -> ("States Out"=w810:string)  [unwired: 13 in]
      }
      frame "Main: HPD Sanity Check" {
        # "Check if gate valve between COMP and M123 is Open"
        n328 = Unbundle By Name(w894) -> ("Chamber Selection.BTL2"=w892:bool, "Chamber Selection.HPD"=w893:bool)
        n329 = case shown="True" w893 {
          tunnel: w899 -> [w902 w910]
          tunnel: w898 -> [_ w909]
          tunnel: [w902 w908] -> w897
          tunnel: w896 -> [_ w907]
          tunnel: ["" w906] -> w895
          tunnel: w894 -> [_ w905]
          tunnel: w892 -> [_ w903]
          tunnel: w891 -> [_ w904]
          frame False {
          }
          frame True {
            # "Check Conditions"
            n330 = case shown="\"False\", Default" w904 {
              selector: w904 -> [_ w916]
              tunnel: w910 -> [w915 w933]
              tunnel: w909 -> [_ w932]
              tunnel: [w915 w930] -> w908
              tunnel: w907 -> [_ w927]
              tunnel: [w911 w921] -> w906
              tunnel: w905 -> [_ w919]
              tunnel: w903 -> [w913 _]
              frame "False", Default {
                # "COMP SELECTED?"
                n331 = Select(t="", s=w913, f="Main: HPD Sanity Check>>BLT2-HPD") -> (s? t:f=w911:string)
              }
              frame "BLT2-HPD" {
                w928 = Error_codes."003-Chamber Gate Valve Status" ("Error Codes")
                # "Event TAG"
                n332 = case shown="\"BLT2-HPD\"" w916 {
                  tunnel: [w935 w936] -> w934
                  frame "False", Default {
                    w935 = T32[] [enum."No Action"] items=["No Action", "Is EC GPM Mode ON?", "Is EC GPM Mode Off?", "Is EC GVM Mode ON?", "Is EC GVM Off?", "Is  EC GPM or GVM Mode ON?", "Is LB GPM Mode ON?", "Is LB GPM Mode Off?", "Is LB GVM Mode ON?", "Is LB GVM Mode Off?", "Is  LB GPM or GVM Mode ON?", "Is M123 Turbo Gate Valve Opened? ", "Is M123 Turbo Gate Valve Closed?", "Is OAP Turbo Gate Valve Opened?", "Is OAP Turbo Gate Valve Closed?", "Is BTLTurbo Gate Valve Opened?", "Is BTL Turbo Gate Valve Closed?", "Is TARGET Turbo Gate Valve 1Opened?", "Is TARGET1 Turbo Gate Valve Closed?", "Is TARGET Turbo Gate Valve 2 Opened?", "Is TAREGT2 Turbo Gate Valve Closed?", "Is BTL2 Turbo Gate Valve Opened?", "Is BTL2 Turbo Gate Valve Closed?", "Is HPD Turbo Gate Valve Opened?", "Is HPD Turbo Gate Valve Closed?", "Is COMP to M123 gate Valve Opened?", "Is COMP to M123 Valve Closed?", "Is HPBD Gate Valve Opened?", "Is HPBD Gate Valve Closed?", "Is M123 to OAP gate valve opened?", "Is M123 to OAP gate valve closed?", "Is OAP to BLT gate valve opened?", "Is OAP to BTL Gate Valve Closed?", "Is BLT to TARGET gate valve opened?", "Is BTL to TARGET Gate Valve Closed?", "Is TARGET to BLT2 gate valve opened?", "Is TARGET to BTL2 Gate Valve Closed?", "Is BLT2 to HPD gate valve opened?", "Is BTL2 to HPD Gate Valve Closed?", "Is COMP at Atmospheric Pressure?", "Is M123 at Atmospheric Pressure?", "Is BeamDump at Atmospheric Pressure?", "Is OAP at Atmospheric Pressure?", "Is BLT at Atmospheric Pressure", "Is TARGET at Atmospheric Pressure?", "Is BLT2 at Atmospheric Pressure?", "Is HPD at Atmospheric Pressure?", "Is the EC Roughing Pump ON?", "Is the EC Roughing Pump OFF?", "Does the EC Roughing Pump have a fault?", "Is the LB Roughing Pump ON?", "Is the LB Roughing Pump Off?", "Does the LB Roughing Pump have a fault?", "Is the EC Backing Pump ON?", "Is the EC Backing Pump OFF?", "Is the LB Backing Pump ON?", "Is the LB Backing Pump OFF?", "Does the EC Backing Pump have a fault?", "Does the LB Backing Pump have a fault?", "Is the EC Backing Pipe at Atmospheric Pressure", "Is the LB Backing Pipe at Atmospheric Pressure", "Is the EC Backing Manifold at Atmospheric Pressure", "s the LB Backing Manifold at Atmospheric Pressure?", "Is the EC Roughing Pipe at Atmospheric Pressure", "Is the LB Roughing Pipe at Atmospheric Pressure?", "Is the EC Roughing Manifold at Atmospheric Pressure", "Is the LB Roughing Manifold at Atmospheric Pressure", "Is LB Backing Manifold Valve Opened?", "Is EC Backing Manifold Valve Opened?", "Is LB Roughing Manifold Valve Opened?", "Is EC Roughing Manifold Valve Opened?", "Is COMP Roughing Valve Opened?", "Is M123 Roughing Valve Opened?", "Is M123 Roughing Valve Closed?", "Is OAP Roughing Valve Opened?", "Is OAP Roughing Valve Closed?", "Is HPBD Roughing Valve Opened?", "Is HPBD Roughing Valve Closed?", "Is BTL Roughing Valve Opened?", "Is BTL Roughing Valve Closed?", "Is TARGET Roughing Valve Opened?", "Is TARGET Roughing Valve Closed?", "Is BTL2 Roughing Valve Opened?", "Is BTL2 Roughing Valve Closed?", "Is HPD Roughing Valve Opened?", "Is HPD Roughing Valve Closed?", "Is COMP Turbo Backing Valve Opened?", "Is M123 Turbo Backing Valve Opened", "Is HPBD Turbo Backing Valve Opened?", "Is OAP Turbo Backing Valve Opened?", "Is BTL Turbo Backing Valve Opened?", "Is TARGET1 Turbo Backing Valve Opened?", "Is TARGET2 Turbo Backing Valve Opened?", "Is BTL2 Turbo Backing Valve Opened?", "Is HPD Turbo Backing Valve Opened?", "Is M123 Backing at MID-VAC?", "Is OAP Backing at MID-VAC?", "Is TARGET1 Backing at MID-VAC?", "Is TARGET2 Backing at MID-VAC?", "Is BTL Backing at MID-VAC?", "Is BTL2 Backing at MID-VAC?", "Is HPD Backing at MID-VAC?", "Is M123 Turbo in Normal Operation", "Is COMP Turbo in Normal Operation", "Is OAP Turbo in Normal Operation", "Is BTL Turbo in Normal Operation", "Is TARGET1 Turbo in Normal Operation", "Is TARGET2 Turbo in Normal Operation", "Is BTL2 Turbo in Normal Operation", "Is HPD Turbo in Normal Operation", "Is M123 at MID-VAC?", "Is OAP at MID-VAC?", "Is COMP at MID-VAC?", "Is BTL at MID-VAC?", "Is TARGET at MID-VAC?", "Is BTL2 at MID-VAC?", "Is HPD at MID-VAC?"]
                  }
                  frame "BLT2-HPD" {
                    w936 = T32[] [enum."Is BTL2 to HPD Gate Valve Closed?"] items=["No Action", "Is EC GPM Mode ON?", "Is EC GPM Mode Off?", "Is EC GVM Mode ON?", "Is EC GVM Off?", "Is  EC GPM or GVM Mode ON?", "Is LB GPM Mode ON?", "Is LB GPM Mode Off?", "Is LB GVM Mode ON?", "Is LB GVM Mode Off?", "Is  LB GPM or GVM Mode ON?", "Is M123 Turbo Gate Valve Opened? ", "Is M123 Turbo Gate Valve Closed?", "Is OAP Turbo Gate Valve Opened?", "Is OAP Turbo Gate Valve Closed?", "Is BTLTurbo Gate Valve Opened?", "Is BTL Turbo Gate Valve Closed?", "Is TARGET Turbo Gate Valve 1Opened?", "Is TARGET1 Turbo Gate Valve Closed?", "Is TARGET Turbo Gate Valve 2 Opened?", "Is TAREGT2 Turbo Gate Valve Closed?", "Is BTL2 Turbo Gate Valve Opened?", "Is BTL2 Turbo Gate Valve Closed?", "Is HPD Turbo Gate Valve Opened?", "Is HPD Turbo Gate Valve Closed?", "Is COMP to M123 gate Valve Opened?", "Is COMP to M123 Valve Closed?", "Is HPBD Gate Valve Opened?", "Is HPBD Gate Valve Closed?", "Is M123 to OAP gate valve opened?", "Is M123 to OAP gate valve closed?", "Is OAP to BLT gate valve opened?", "Is OAP to BTL Gate Valve Closed?", "Is BLT to TARGET gate valve opened?", "Is BTL to TARGET Gate Valve Closed?", "Is TARGET to BLT2 gate valve opened?", "Is TARGET to BTL2 Gate Valve Closed?", "Is BLT2 to HPD gate valve opened?", "Is BTL2 to HPD Gate Valve Closed?", "Is COMP at Atmospheric Pressure?", "Is M123 at Atmospheric Pressure?", "Is BeamDump at Atmospheric Pressure?", "Is OAP at Atmospheric Pressure?", "Is BLT at Atmospheric Pressure", "Is TARGET at Atmospheric Pressure?", "Is BLT2 at Atmospheric Pressure?", "Is HPD at Atmospheric Pressure?", "Is the EC Roughing Pump ON?", "Is the EC Roughing Pump OFF?", "Does the EC Roughing Pump have a fault?", "Is the LB Roughing Pump ON?", "Is the LB Roughing Pump Off?", "Does the LB Roughing Pump have a fault?", "Is the EC Backing Pump ON?", "Is the EC Backing Pump OFF?", "Is the LB Backing Pump ON?", "Is the LB Backing Pump OFF?", "Does the EC Backing Pump have a fault?", "Does the LB Backing Pump have a fault?", "Is the EC Backing Pipe at Atmospheric Pressure", "Is the LB Backing Pipe at Atmospheric Pressure", "Is the EC Backing Manifold at Atmospheric Pressure", "s the LB Backing Manifold at Atmospheric Pressure?", "Is the EC Roughing Pipe at Atmospheric Pressure", "Is the LB Roughing Pipe at Atmospheric Pressure?", "Is the EC Roughing Manifold at Atmospheric Pressure", "Is the LB Roughing Manifold at Atmospheric Pressure", "Is LB Backing Manifold Valve Opened?", "Is EC Backing Manifold Valve Opened?", "Is LB Roughing Manifold Valve Opened?", "Is EC Roughing Manifold Valve Opened?", "Is COMP Roughing Valve Opened?", "Is M123 Roughing Valve Opened?", "Is M123 Roughing Valve Closed?", "Is OAP Roughing Valve Opened?", "Is OAP Roughing Valve Closed?", "Is HPBD Roughing Valve Opened?", "Is HPBD Roughing Valve Closed?", "Is BTL Roughing Valve Opened?", "Is BTL Roughing Valve Closed?", "Is TARGET Roughing Valve Opened?", "Is TARGET Roughing Valve Closed?", "Is BTL2 Roughing Valve Opened?", "Is BTL2 Roughing Valve Closed?", "Is HPD Roughing Valve Opened?", "Is HPD Roughing Valve Closed?", "Is COMP Turbo Backing Valve Opened?", "Is M123 Turbo Backing Valve Opened", "Is HPBD Turbo Backing Valve Opened?", "Is OAP Turbo Backing Valve Opened?", "Is BTL Turbo Backing Valve Opened?", "Is TARGET1 Turbo Backing Valve Opened?", "Is TARGET2 Turbo Backing Valve Opened?", "Is BTL2 Turbo Backing Valve Opened?", "Is HPD Turbo Backing Valve Opened?", "Is M123 Backing at MID-VAC?", "Is OAP Backing at MID-VAC?", "Is TARGET1 Backing at MID-VAC?", "Is TARGET2 Backing at MID-VAC?", "Is BTL Backing at MID-VAC?", "Is BTL2 Backing at MID-VAC?", "Is HPD Backing at MID-VAC?", "Is M123 Turbo in Normal Operation", "Is COMP Turbo in Normal Operation", "Is OAP Turbo in Normal Operation", "Is BTL Turbo in Normal Operation", "Is TARGET1 Turbo in Normal Operation", "Is TARGET2 Turbo in Normal Operation", "Is BTL2 Turbo in Normal Operation", "Is HPD Turbo in Normal Operation", "Is M123 at MID-VAC?", "Is OAP at MID-VAC?", "Is COMP at MID-VAC?", "Is BTL at MID-VAC?", "Is TARGET at MID-VAC?", "Is BTL2 at MID-VAC?", "Is HPD at MID-VAC?"]
                  }
                }
                n333 = call "GetAction.vi"("Check Condition"=w928, "Query Array"=w934, "error in (no error)"=w933) -> ("Status Array Out"=w929:string[], "Generate Event?"=w920:bool, "error out"=w931:errorcluster)  [unwired: 7 in, 3 out]
                n334 = Unbundle By Name(w919) -> ("VI Refnum"=w923:refnum<vi>)
                n335 = call "Generate User Event.vi"("Add(t)/Remove(f) Event"=w920, "error in (no error)"=w931, "User Event in"=w932, "Status Array In"=w929, "Error Codes"=w928) -> ("error out"=w930:errorcluster)  [unwired: 5 in, 1 out]
                n336 = Not A Number/Path/Refnum?(number/path/refnum=w923) -> (NaN/Path/Refnum?=w922:bool)
                n337 = case shown="True" w920 {
                  tunnel: ["" w951] -> w921
                  tunnel: w923 -> [w940 w950]
                  tunnel: w922 -> [w941 w949]
                  tunnel: w916 -> [_ w948]
                  frame False {
                    n338 = case shown="True" w941 {
                      tunnel: w940 -> [_ w944]
                      frame False {
                      }
                      frame True {
                        n339 = invoke class="VI" method="Abort VI"(reference=w944) -> (reference out=w942:refnum<vi>, error out=w943:errorcluster)  [unwired: 2 in, 1 out]
                        n340 = case shown="No Error" w943 {
                          selector: w943 -> [w946 _]
                          tunnel: w942 -> [w947 _]
                          frame No Error {
                            n341 = Close Reference(reference=w947, error in (no error)=w946) -> (error out=w945:errorcluster)
                            n342 = invoke on="User Input Panel" class="SubPnl" method="Remove VI"(error in=w945) -> ()  [unwired: 2 in, 3 out]
                          }
                          frame Error {
                          }
                        }
                      }
                    }
                    n343 = call "MID-VAC Timer.vi"("TO sec (Start timer)"=1.0, "Action"=timerAction_typdef."Start Timer") -> ()  [unwired: 9 in, 1 out]
                  }
                  frame True {
                    # "when to is true\nand"
                    n344 = case shown="False" w949 {
                      tunnel: w950 -> [w956 _]
                      tunnel: [w954 w971] -> w951
                      tunnel: w948 -> [w952 w972]
                      frame False {
                        n345 = call "FindControlByName_VEPS.vi"("control name"="Op Out", "vi refnum"=w956) -> ("control refnum"=w958:refnum<vi>)  [unwired: 2 in, 1 out]
                        n346 = property class="Ctl"(reference=w958) -> ("Value"=w957:variant)  [unwired: 1 in, 2 out]
                        n347 = Variant To Data(type=op_typdef."Idle" ("Op Out"), Variant=w957) -> (data=w955:T24)  [unwired: 1 in, 1 out]
                        n348 = case shown="\"Idle\", Default" w955 {
                          tunnel: [w960 w966 "Idle\nMacro: Exit"] -> w954
                          tunnel: w952 -> [w961 w965 _]
                          frame "Idle", Default {
